vi "TCP IP Read.vi"(8 "error in (no error)":errorcluster, 11 "TCP Network Connection in":refnum<k5>) -> (0 "error out":errorcluster, 3 "Data Out":i32[](array[numeric]))   [LabVIEW 2017]
panel:
  out "connection ID out":refnum<k5>
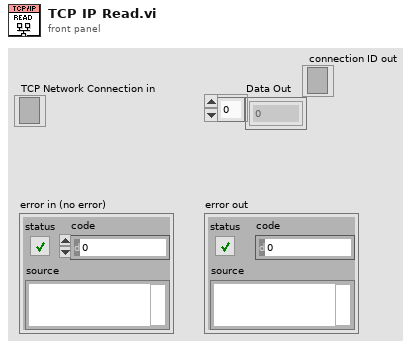
[diagram p1: front panel]
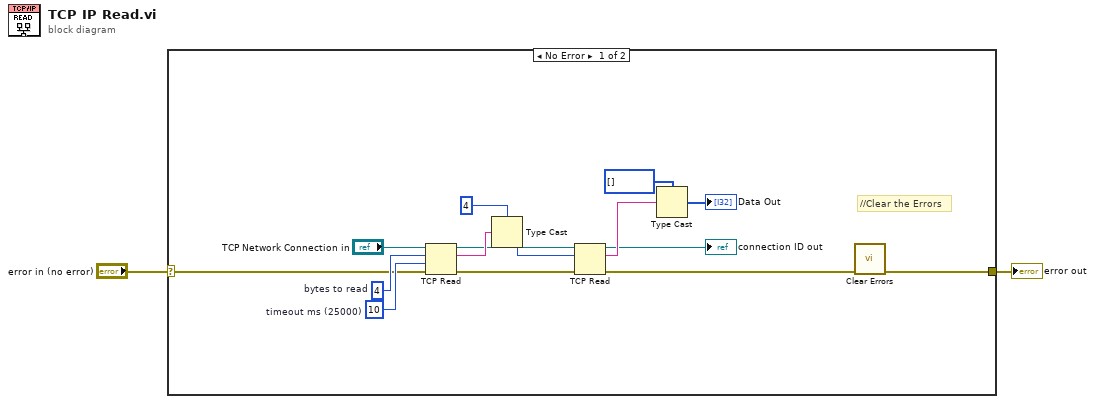
[diagram p0: block diagram]
diagram:
  n1 = case shown="No Error" "error in (no error)" {
    selector: "error in (no error)" -> [w5 w18]
    tunnel: [w3 w18] -> w1
    frame No Error {
      w8 = 4  # bytes to read
      w9 = 10  # timeout ms (25000)
      # "//Clear the Errors"
      n2 = TCP Read(connection ID="TCP Network Connection in", bytes to read=w8, error in (no error)=w5, 9:w9) -> (connection ID out=w10:refnum<k5>, data out=w14:string, error out=w11:errorcluster)  [unwired: 1 in]
      n3 = Type Cast(type=4 ("bytes to read"), x=w14) -> (*(type *) &x=w15:i32)
      n4 = TCP Read(connection ID=w10, bytes to read=w15, error in (no error)=w11) -> (connection ID out=→"connection ID out":refnum<k5>, data out=w12:string, error out=w4:errorcluster)  [unwired: 2 in]
      n5 = Type Cast(type=i32[] [], x=w12) -> (*(type *) &x=→"Data Out":i32[])
      n6 = call <vilib>:"Clear Errors.vi"("error in (no error)"=w4) -> ("error out"=w3:errorcluster)  [unwired: 5 in, 1 out]
    }
    frame Error {
    }
  }
  "error out" <- w1
